vi "Read Required.vi"(8 "error in (no error)":errorcluster, 11 "Option in":refnum<class "Option.lvclass">) -> (0 "error out":errorcluster, 2 "Required":bool, 3 "Option out":refnum<class "Option.lvclass">)   [LabVIEW 2011, in "Option Parser.lvlib" / "Option.lvclass"]
uses:
  Option.lvclass
  Option.lvclass/Option.ctl
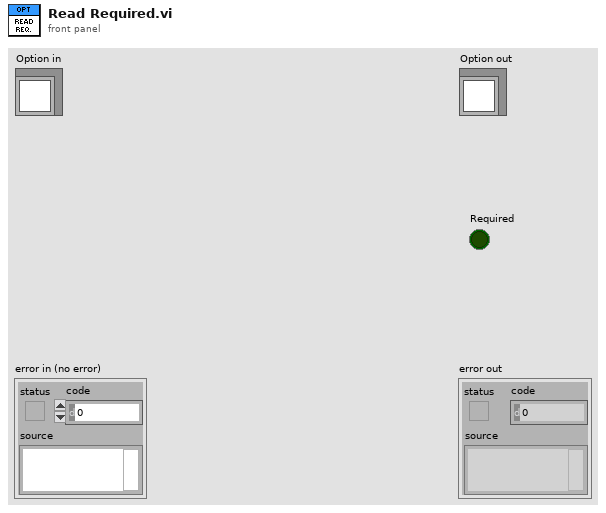
[diagram p1: front panel]
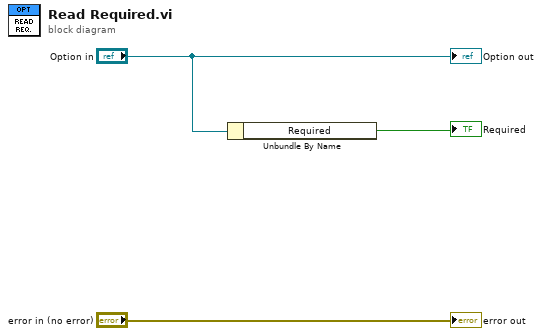
[diagram p0: block diagram]
diagram:
  n1 = Unbundle By Name("Option in") -> ("Required"=→"Required":bool)
  "error out" <- "error in (no error)"
  "Option out" <- "Option in"
